vi "Load Config.vi"(8 "error in (no error)":errorcluster, 11 "DigitalOutChannel in":refnum<class "DigitalOutChannel.lvclass">) -> (0 "error out":errorcluster, 3 "DigitalOutChannel out":refnum<class "DigitalOutChannel.lvclass">)   [LabVIEW 2020, in "VolatusDAQConfig.lvlib" / "DigitalOutChannel.lvclass"]
uses:
  DigitalOutChannel.lvclass
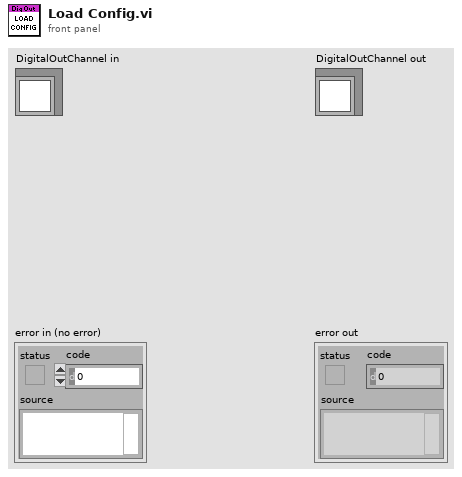
[diagram p1: front panel]
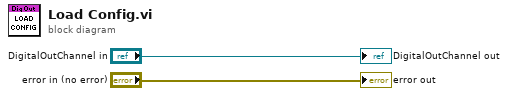
[diagram p0: block diagram]
diagram:
  "error out" <- "error in (no error)"
  "DigitalOutChannel out" <- "DigitalOutChannel in"
